vi "CustomErrorManagerConfigure.vi"() -> ()   [LabVIEW 2021]
uses:
  ErrorCreationExecution/ErrorCreationExecution.lvclass
panel:
  in  "Cancel":bool
  in  "OK":bool
  in  "End of Range":i32
  in  "Start of Range":i32
  in  "Default Error Handler":u16(ring) items=["ErrorCreationJSON.lvclass", "ErrorCreationMGI.lvclass"]
  in  "Database File Path":path
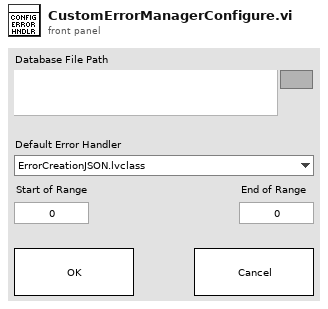
[diagram p1: front panel]
types:
  T1 = typedef "ConfigurationData.ctl" = cluster{"DataSetFilePath":path, "DefaultErrorCreationType":string, "StartOfErrorRange":i32, "EndOfErrorRange":i32, "FirstUse":bool}
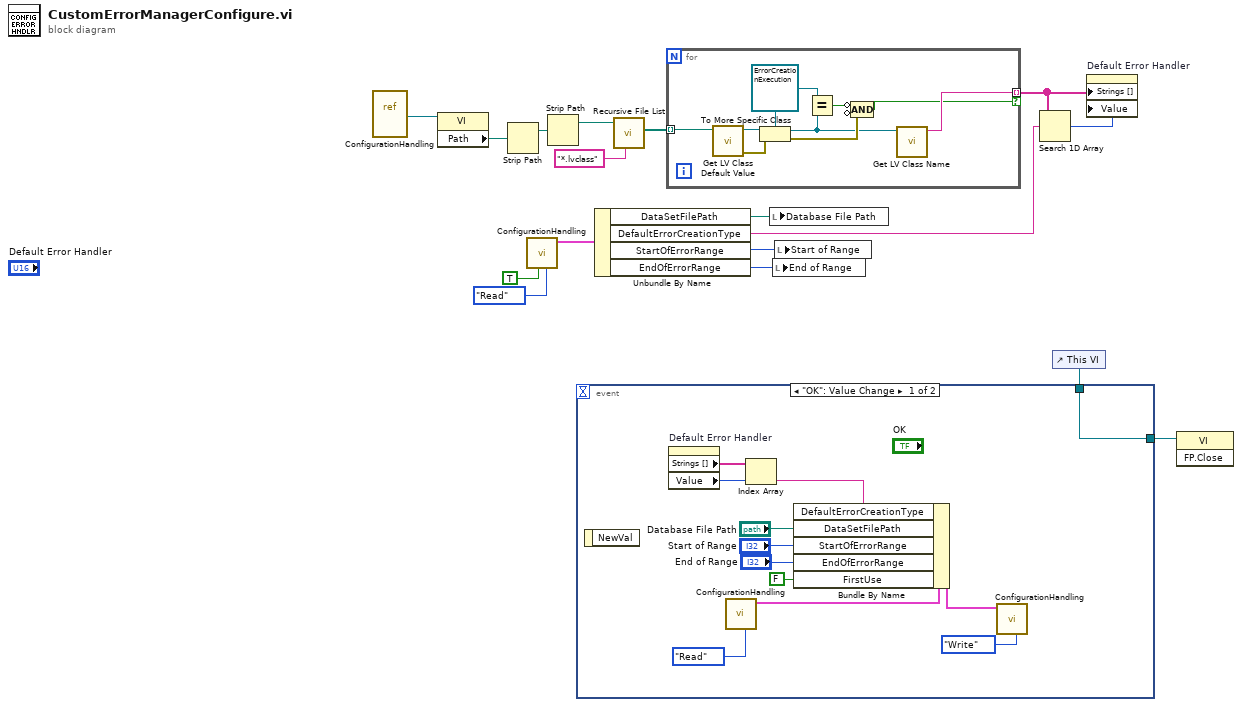
[diagram p0: block diagram]
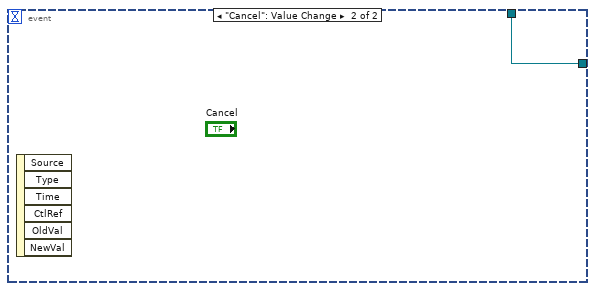
[diagram p2: hidden frame]
diagram:
  n1 = vi-ref "ConfigurationHandling.vi"() -> (w13:refnum<vi>)
  n2 = property class="VI"(reference=w13) -> ("Path"=w12:path)  [unwired: 1 in, 2 out]
  n3 = Strip Path(path=w12) -> (stripped path=w11:path)  [unwired: 1 out]
  n4 = call "ConfigurationHandling.vi"("Function"=enum16{"Read", "Write"}."Read", "ForceReload"=TRUE) -> ("SettingsOut"=w15:T1)  [unwired: 9 in]
  n5 = Strip Path(path=w11) -> (stripped path=w10:path)  [unwired: 1 out]
  n6 = Unbundle By Name(w15) -> ("DataSetFilePath"=w14:path, "DefaultErrorCreationType"=w6:string, "StartOfErrorRange"=w3:i32, "EndOfErrorRange"=w4:i32)
  n7 = call <vilib>:"Recursive File List.vi"("pattern"="*.lvclass", "Folder Path"=w10) -> ("All Files in Dir"=w8:path[])  [unwired: 5 in, 4 out]
  n8 = for {
    tunnel: w8 -> [w26] mode=indexing
    tunnel: [w19] -> w7 mode=indexing if=w18
    w23 = refnum<class "ErrorCreationExecution.lvclass"> refnum ("ErrorCreationExecution")
    n9 = call <vilib>:"Get LV Class Default Value.vi"("class path"=w26) -> ("error out"=w25:errorcluster, "object"=w24:refnum<class>)  [unwired: 9 in]
    n10 = To More Specific Class(target class=w23, reference=w24, error in=w25) -> (specific class reference=w20:refnum<class "ErrorCreationExecution.lvclass">, error out=w21:errorcluster)
    n11 = Equal?(x=w23, y=w20) -> (x = y?=w22:bool)
    n12 = Compound Arithmetic op=AND(invert w22, invert w21) -> (w18:bool)
    n13 = call <vilib>:"Get LV Class Name.vi"("object"=w20) -> ("class name"=w19:string)  [unwired: 9 in, 1 out]
  }
  n14 = local write "Database File Path"(w14) -> ()
  n15 = local write "End of Range"(w4) -> ()
  n16 = local write "Start of Range"(w3) -> ()
  n17 = Search 1D Array(1D array=w7, element=w6) -> (index of element=w5:i32)  [unwired: 1 in]
  n18 = control-ref of="This VI"() -> (w1:refnum<vi>)
  n19 = event shown="[0] \"OK\": Value Change" {
    selector: _ -> [_ _]
    dyn-events: _ -> [_ _]
    timeout: _ -> [_ _]
    tunnel: [w27 w39] -> w2
    tunnel: w1 -> [w27 w39]
    event "OK": Value Change {
      n20 = event-data() -> ()  [unwired: 1 in, 1 out]
      n21 = property on="Default Error Handler" class="Ring (strict)"() -> ("Strings []"=w32:string[], "Value"=w33:u16)  [unwired: 2 in, 2 out]
      n22 = call "ConfigurationHandling.vi"("Function"=enum16{"Read", "Write"}."Read") -> ("SettingsOut"=w37:T1)  [unwired: 10 in]
      n23 = Index Array(array=w32, index=w33) -> (element=w31:string)
      n24 = Bundle By Name(cluster=w37, "DefaultErrorCreationType"=w31, "DataSetFilePath"="Database File Path", "StartOfErrorRange"="Start of Range", "EndOfErrorRange"="End of Range", "FirstUse"=FALSE) -> (w29:T1)
      n25 = call "ConfigurationHandling.vi"("Function"=enum16{"Read", "Write"}."Write", "SettingsIn"=w29) -> ()  [unwired: 9 in, 1 out]
    }
    event "Cancel": Value Change {
      n26 = event-data() -> ()  [unwired: 1 in, 6 out]
    }
  }
  n27 = property on="Default Error Handler" class="Ring (strict)"("Strings []"=w7, "Value"=w5) -> ()  [unwired: 2 in, 2 out]
  n28 = invoke class="VI" method="FP.Close"(reference=w2) -> ()  [unwired: 2 in, 3 out]
